vi "test Read U32 Array.vi"(8 "error in (no error)":errorcluster, 11 "TestCase in":refnum<class "Buffer Tests.lvclass">=refnum) -> (0 "error out":errorcluster, 3 "TestCase out":refnum<class "Buffer Tests.lvclass">)   [LabVIEW 2021, in "Buffer Tests.lvclass"]
uses:
  Buffer Tests.lvclass
  Classes/Buffer/Buffer.lvclass
  <vilib>/NI/Memory Manager/Classes/Pointer/Pointer.lvclass
  Classes/Buffer/Read Buffer 1D U32.vi
  C:/Program Files/National Instruments/LabVIEW 2021/vi.lib/NI/Memory Manager/Classes/Pointer/Pointer.lvclass
  C:/dev/git/custom-devices/niveristand-data-sharing-framework-custom-device/Source/Core/Classes/Buffer/Buffer.lvclass
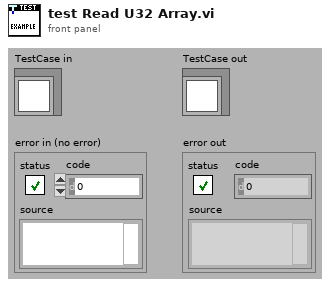
[diagram p1: front panel]
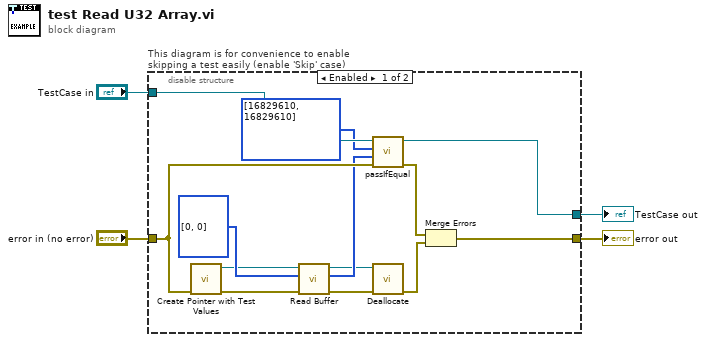
[diagram p0: block diagram]
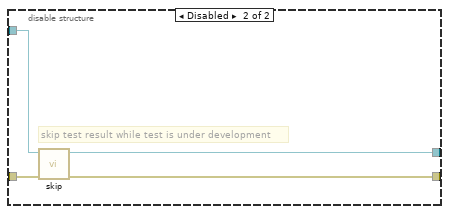
[diagram p2: hidden frame]
diagram:
  n1 = disable-structure "This diagram is for convenience to enable skipping a test easily (enable 'Skip' case)" shown="Enabled" {
    disable-tunnel: "TestCase in" -> [w14 w21]
    disable-tunnel: [w15 w19] -> w1
    disable-tunnel: [w12 w20] -> w2
    disable-tunnel: "error in (no error)" -> [w13 w18]
    frame Enabled {
      n2 = call "Create Pointer with Test Values.vi"("error in (no error)"=w13) -> ("error out"=w8:errorcluster, "Buffer out"=w7:refnum<class "Buffer.lvclass">)  [unwired: 9 in]
      n3 = call-poly "Read Buffer.vi"("error in (no error)"=w8, "dst array in"=u32[] [0, 0] ("buffer in"), "Buffer in"=w7) -> ("error out"=w17:errorcluster, "dst array out"=w10:u32[], "Buffer out"=w5:refnum<class "Buffer.lvclass">)  [unwired: 5 in, 1 out]
      n4 = call-dynamic "passIfEqual.vi"("error in (no error)"=w13, "y"=w10, "x"=u32[] [16829610, 16829610] ("reversed array 3"), "TestCase in"=w14) -> ("error out"=w16:errorcluster, "TestCase out"=w15:refnum<class "Buffer Tests.lvclass">)  [unwired: 6 in]
      n5 = call <vilib>:"Deallocate.vi"("error in (no error)"=w17, "Pointer"=w5) -> ("error out"=w6:errorcluster)  [unwired: 8 in, 1 out]
      n6 = Merge Errors(w16, w6) -> (w12:errorcluster)
    }
    frame Disabled {
      # "skip test result while test is under development"
      n7 = call <vilib>:"skip.vi"("error in (no error)"=w18, "TestCase in"=w21) -> ("error out"=w20:errorcluster, "TestCase out"=w19:refnum<class "Buffer Tests.lvclass">)  [unwired: 8 in]
    }
  }
  "error out" <- w2
  "TestCase out" <- w1
